vi "trip.vi"(10 "Trip":dbl, 11 "Array":T1[](array[typedef]) {"Data" format="%.0x"}) -> (3 "Array 2":T1[](array[typedef]) {"Data" format="%.0x"})   [LabVIEW 2021, in "uCanDriver.lvlib" / "uCAN.lvclass"]
uses:
  uCAN.lvclass
  typedefs/frame.ctl
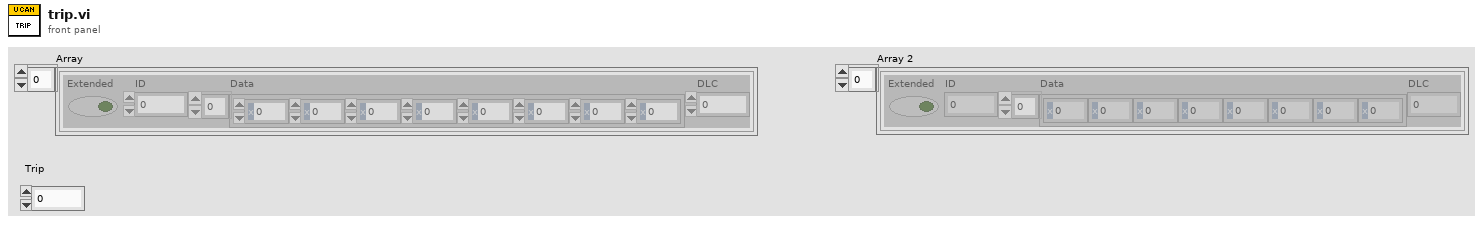
[diagram p1: front panel]
types:
  T1 = typedef "uCanDriver.lvlib/uCAN.lvclass/frame.ctl" = cluster{"Extended":bool, "ID":u32, "Data":u8[], "DLC":u8}
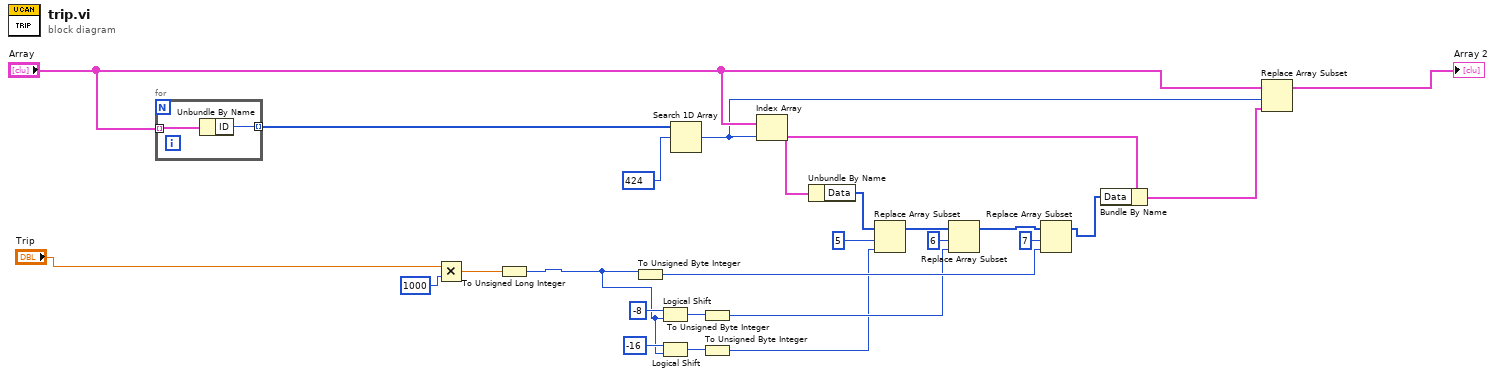
[diagram p0: block diagram]
diagram:
  n1 = for {
    tunnel: "Array" -> [w27] mode=indexing
    tunnel: [w26] -> w23 mode=indexing
    n2 = Unbundle By Name(w27) -> ("ID"=w26:u32)
  }
  n3 = Multiply(x="Trip", y=i16 1000) -> (x*y=w2:dbl)
  n4 = To Unsigned Long Integer(number=w2) -> (unsigned 32bit integer=w1:u32)
  n5 = To Unsigned Byte Integer(number=w1) -> (unsigned 8bit integer=w5:u8)
  n6 = Logical Shift(y=i16 -8, x=w1) -> (x << y=w13:u32)
  n7 = Logical Shift(y=i16 -16, x=w1) -> (x << y=w7:u32)
  n8 = Search 1D Array(1D array=w23, element=u32 424) -> (index of element=w21:i32)  [unwired: 1 in]
  n9 = To Unsigned Byte Integer(number=w13) -> (unsigned 8bit integer=w4:u8)
  n10 = To Unsigned Byte Integer(number=w7) -> (unsigned 8bit integer=w3:u8)
  n11 = Index Array(array="Array", index=w21) -> (element=w25:T1)
  n12 = Unbundle By Name(w25) -> ("Data"=w17:u8[])
  n13 = Replace Array Subset(array=w17, new element=w3, index=5) -> (w16:u8[])
  n14 = Replace Array Subset(array=w16, new element=w4, index=6) -> (w8:u8[])
  n15 = Replace Array Subset(array=w8, new element=w5, index=7) -> (w9:u8[])
  n16 = Bundle By Name(cluster=w25, "Data"=w9) -> (w19:T1)
  n17 = Replace Array Subset(array="Array", new element=w19, index=w21) -> (→"Array 2":T1[])
